vi "TrapezoidProfile_Position_Control_Example.vi"() -> ()   [LabVIEW 2019]
uses:
  <vilib>/Rock Robotics/WPI/ThirdParty/JAS_Junk/TrajLib/TrapProfile_Calculate.vi
  <vilib>/Rock Robotics/WPI/ThirdParty/JAS_Junk/TrajLib/TrapProfile_New.vi
  <vilib>/Rock Robotics/WPI/ThirdParty/JAS_Junk/TrajLib/TrapProfile_TotalTime.vi
  <vilib>/Rock Robotics/WPI/ThirdParty/JAS_Junk/TrajLib/TrapProfConstraint_New.vi
  <vilib>/Rock Robotics/WPI/ThirdParty/JAS_Junk/TrajLib/TrapProfState_New.vi
  <vilib>/Rock Robotics/WPI/ThirdParty/JAS_Junk/TrajLib/TrapProfile_IsFinished.vi
  <vilib>/Rock Robotics/WPI/ThirdParty/JAS_Junk/TrajLib/SimpleMotorFF_Calculate.vi
  <vilib>/Rock Robotics/WPI/ThirdParty/JAS_Junk/TrajLib/TrapProfile_Direct.vi
  <vilib>/Rock Robotics/WPI/ThirdParty/JAS_Junk/TrajLib/TrapProfile_ShouldFlipAcceleration.vi
  <vilib>/Rock Robotics/SystemInterfaces/NetworkCommunication/NetComm_UsageReport_report.vi
  <vilib>/Rock Robotics/WPI/ThirdParty/JAS_Junk/TrajLib/Util_LibraryGlobals.vi
  <vilib>/Rock Robotics/WPI/ThirdParty/JAS_Junk/TrajLib/Trajectory_Library.lvlib
panel:
  in  "Tab Control":T1(tab)
  out "Speed Chart":T2(graph)
  in  "Desired Position\nFt":dbl(slide) min=0.0 max=90.0 scale=-50.0..50.0
  in  "Set Desired \nPosition to \n0 Ft":bool
  in  "Set Desired \nPosition to\n15 ft":bool
  in  "Turn on to\nuse slider\nas setpoint":bool
  out "Position Error":dbl format="%14.2f"
  out "SP, PV, CO Chart":T3(graph)
  out "In Position":bool
  out "Motor-Demand":dbl format="%14.3f"
  out "Position\nFt":dbl format="%14.2f"
  out "Setpoint\nFt":dbl format="%14.2f"
  out "Velocity Ft/Sec":dbl format="%16.1f"
  out "Velocity SP Ft/Sec":dbl format="%16.1f"
  in  "Max Accel":dbl=7.0 format="%#_13g"
  # "Example of Using Trapezoid Profile for Position Control"
  # "Simulate a robot driving forward to a particular position.  A function generator is used to calculate the desired\nmotor output based on the position error.  The maximum robot speed is 8 ft/sec."
  # "Press one of the buttons \nto set the desired position.  \nThis \"target\" value is \ncalledthe \"Set Point\"."
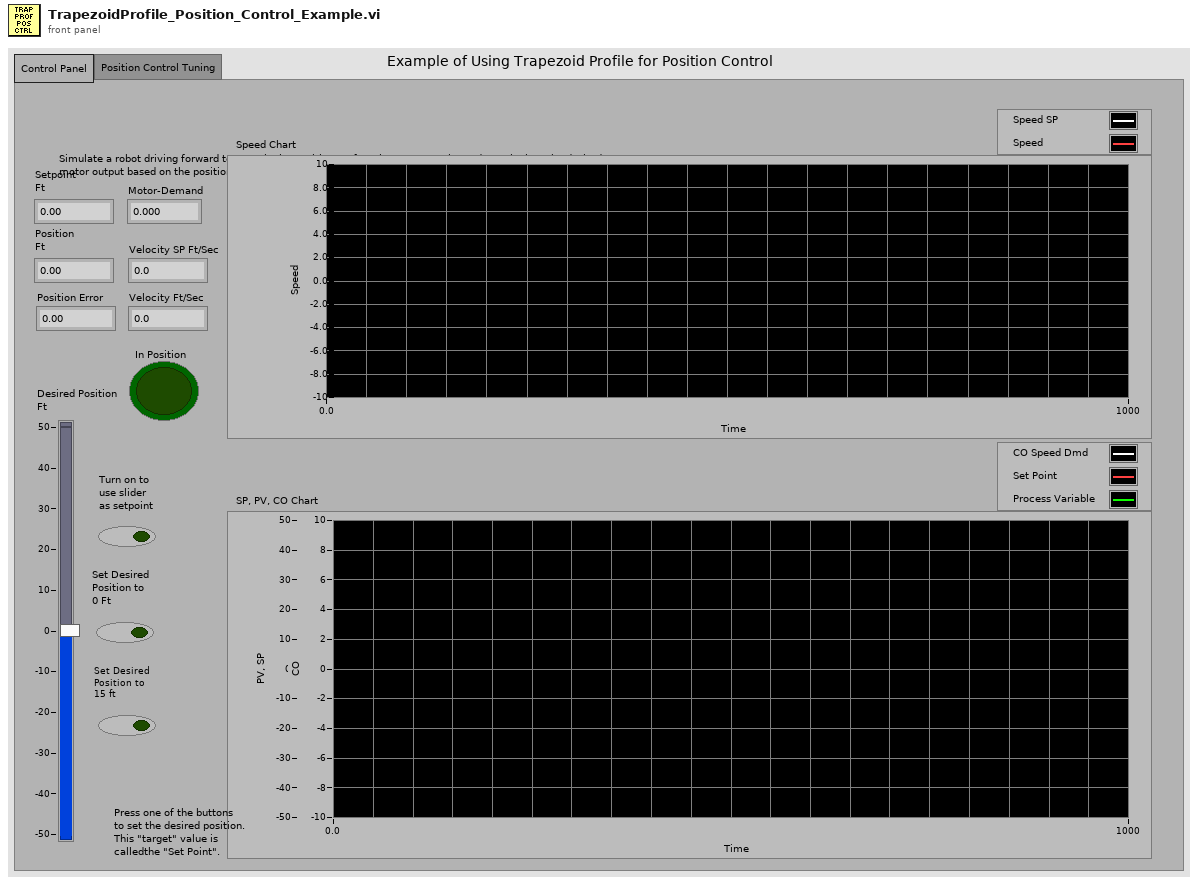
[diagram p1: front panel]
types:
  T1 = enum32{"Control Panel", "Position Control Tuning"}
  T2 = cluster{"Velocity SP Ft/Sec":dbl, "Velocity Ft/Sec":dbl}
  T3 = cluster{"MotorDemand":dbl, "CurrentSetpoint":dbl, "CurrentPosition":dbl}
  T4 = cluster{"Velocity SP Ft/Sec":dbl, "Setpoint\nFt":dbl, "Position\nFt":dbl}
  T5 = typedef "Trajectory_Library.lvlib/SIMPLE_MOTOR_FF.ctl" = cluster{"Ks":dbl, "Kv":dbl, "Ka":dbl, "KnInv":dbl}
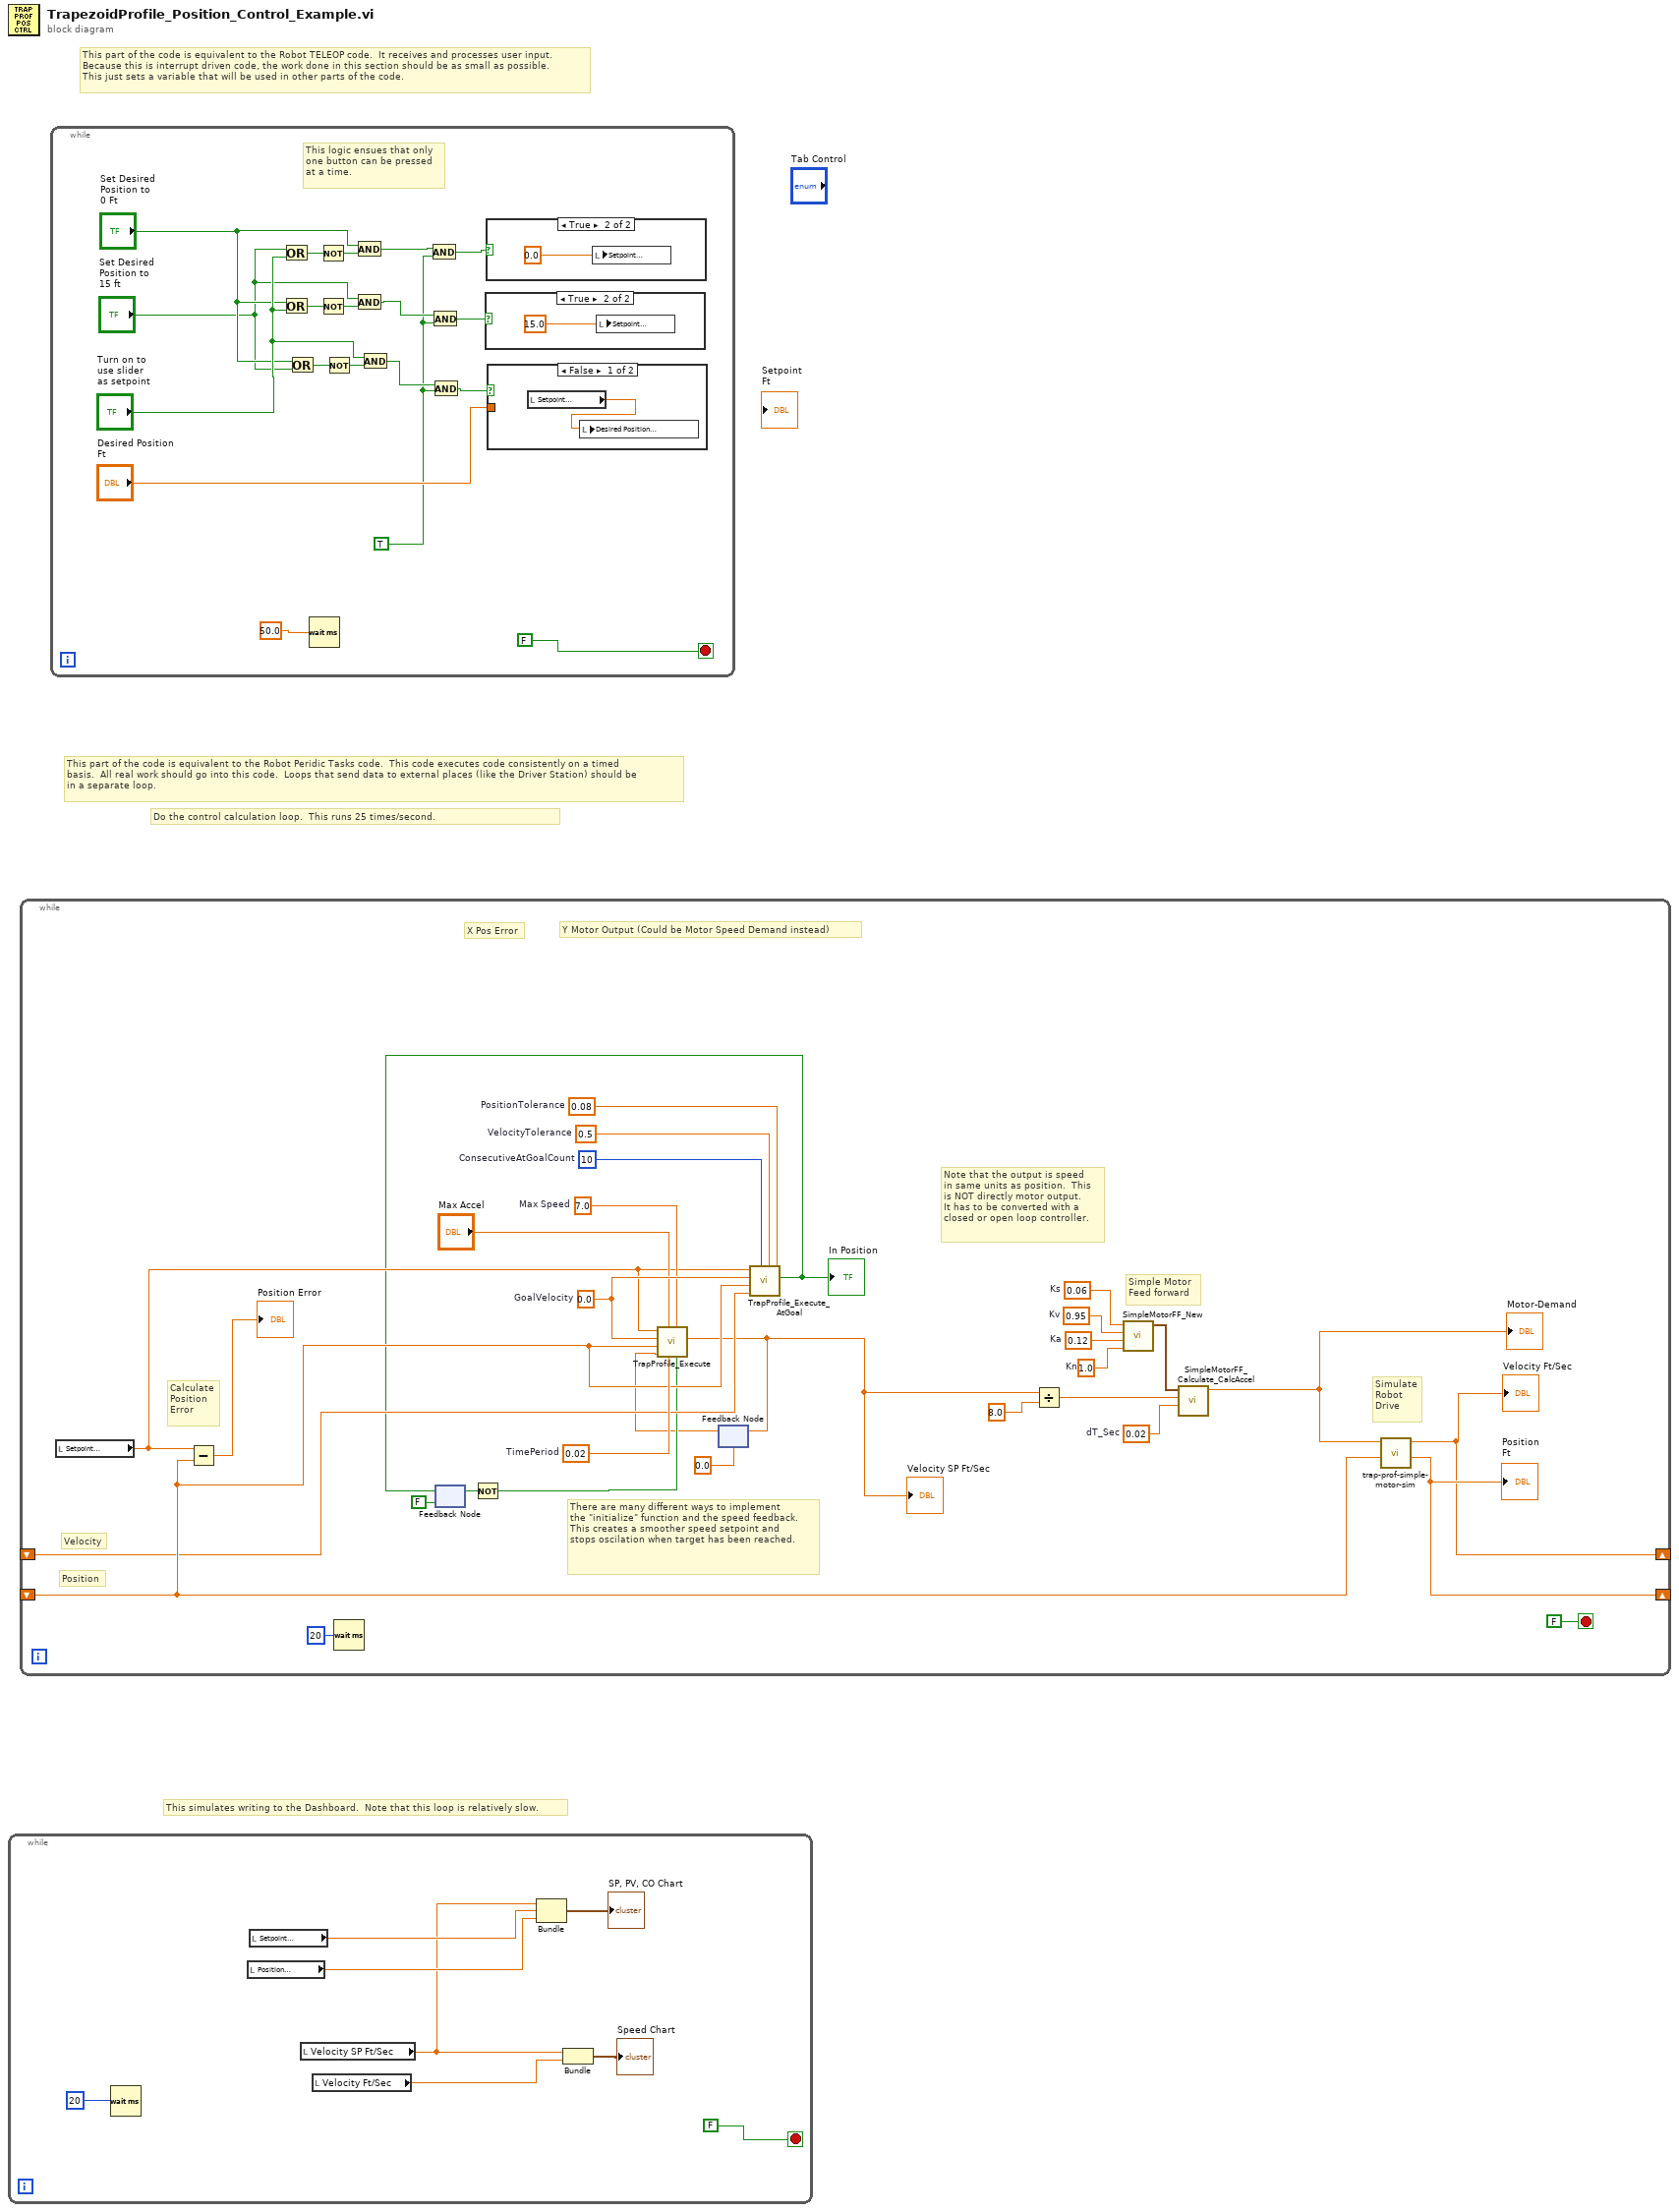
[diagram p0: block diagram]
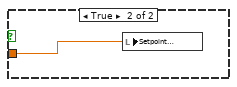
[diagram p2: hidden frame]
diagram:
  # "This simulates writing to the Dashboard.  Note that this loop is relatively slow."
  # "Do the control calculation loop.  This runs 25 times/second."
  # "This part of the code is equivalent to the Robot Peridic Tasks code.  This code executes code consistently on a timed\nbasis.  All real work should go into this code.  Loops that send data to external places (like the Driver Station) should be \nin a separate loop."
  # "This part of the code is equivalent to the Robot TELEOP code.  It receives and processes user input.\nBecause this is interrupt driven code, the work done in this section should be as small as possible.\nThis just sets a variable that will be used in other parts of the code."
  n1 = while {
    stop <- FALSE stop-if-true
    n2 = Wait (ms)(milliseconds to wait=u32 20) -> ()  [unwired: 1 out]
    n3 = local read "Position\nFt"() -> (w4:dbl)
    n4 = local read "Setpoint\nFt"() -> (w6:dbl)
    n5 = local read "Velocity SP Ft/Sec"() -> (w1:dbl)
    n6 = local read "Velocity Ft/Sec"() -> (w3:dbl)
    n7 = Bundle("Velocity SP Ft/Sec"=w1, "Setpoint\nFt"=w6, "Position\nFt"=w4) -> (→"SP, PV, CO Chart":T4)  [unwired: 1 in]
    n8 = Bundle("Velocity SP Ft/Sec"=w1, "Velocity Ft/Sec"=w3) -> (→"Speed Chart":T2)  [unwired: 1 in]
  }
  n9 = while {
    shift-right: [w37] -> _
    shift-left: _ -> [w28]
    shift-right: [w29] -> _
    shift-left: _ -> [w27]
    stop <- FALSE stop-if-true
    w24 = 1.0  # Kn
    w23 = 0.02  # dT_Sec
    w21 = 0.06  # Ks
    w20 = 0.95  # Kv
    w19 = 0.12  # Ka
    w34 = 10  # ConsecutiveAtGoalCount
    w35 = 0.5  # VelocityTolerance
    w36 = 0.08  # PositionTolerance
    w33 = 0.0  # GoalVelocity
    w31 = 0.02  # TimePeriod
    w32 = 7.0  # Max Speed
    # "Velocity"
    # "Position"
    # "Simple Motor\nFeed forward"
    # "Note that the output is speed\nin same units as position.  This\nis NOT directly motor output.\nIt has to be converted with a \nclosed or open loop controller."
    # "There are many different ways to implement\nthe \"initialize\" function and the speed feedback.\nThis creates a smoother speed setpoint and\nstops oscilation when target has been reached."
    # "Y Motor Output (Could be Motor Speed Demand instead)"
    # "X Pos Error"
    # "Calculate\nPosition\nError"
    # "Simulate\nRobot\nDrive"
    n10 = local read "Setpoint\nFt"() -> (w25:dbl)
    n11 = Subtract(x=w25, y=w28) -> (x-y=→"Position Error":dbl)
    n12 = Wait (ms)(milliseconds to wait=u32 20) -> ()  [unwired: 1 out]
    n13 = feedback #1(FALSE ("AtGoal")) -> (w14:bool)
    n14 = Not(x=w14) -> (.not. x?=w13:bool)
    n15 = feedback #2(0.0 ("VelocityDmd")) -> (w11:dbl)
    n16 = call <vilib>:"TrapProfile_Execute.vi"("Initialize"=w13, "Max Speed"=w32, "TimePeriod"=w31, "Max Accel"="Max Accel", "CurrentVelocity"=w11, "CurrentPosition"=w28, "GoalVelocity"=w33, "GoalPosition"=w25) -> ("VelocityDmd"=w12:dbl)  [unwired: 3 out]
    "Velocity SP Ft/Sec" <- w12
    n17 = feedback-in #2(w12) -> ()
    n18 = call <vilib>:"TrapProfile_Execute_AtGoal.vi"("PositionTolerance"=w36, "VelocityTolerance"=w35, "ConsecutiveAtGoalCount"=w34, "CurrentVelocity"=w27, "CurrentPosition"=w28, "GoalVelocity"=w33, "GoalPosition"=w25) -> ("AtGoal"=w16:bool)  [unwired: 4 in]
    "In Position" <- w16
    n19 = feedback-in #1(w16) -> ()
    n20 = Divide(x=w12, y=8.0) -> (x/y=w18:dbl)
    n21 = call <vilib>:"SimpleMotorFF_New.vi"("Kn"=w24, "Ka"=w19, "Kv"=w20, "Ks"=w21) -> ("SIMPLE_MOTOR_FF"=w22:T5)  [unwired: 7 in]
    n22 = call <vilib>:"SimpleMotorFF_Calculate_CalcAccel.vi"("dT_Sec"=w23, "VelSp"=w18, "SIMPLE_MOTOR_FF"=w22) -> ("FeedForward"=w17:dbl)  [unwired: 8 in]
    "Motor-Demand" <- w17
    n23 = call "trap-prof-simple-motor-sim.vi"("Current Position Ft"=w28, "Motor-Demand"=w17) -> ("Updated Position Ft"=w37:dbl, "Velocity Ft/Sec"=w29:dbl)  [unwired: 8 in]
    "Position\nFt" <- w37
    "Velocity Ft/Sec" <- w29
  }
  n24 = while {
    stop <- FALSE stop-if-true
    w40 = TRUE
    # "This logic ensues that only\none button can be pressed\nat a time."
    n25 = Or(x="Set Desired \nPosition to\n15 ft", y="Turn on to\nuse slider\nas setpoint") -> (x .or. y?=w58:bool)
    n26 = Or(x="Set Desired \nPosition to \n0 Ft", y="Turn on to\nuse slider\nas setpoint") -> (x .or. y?=w56:bool)
    n27 = Or(x="Set Desired \nPosition to \n0 Ft", y="Set Desired \nPosition to\n15 ft") -> (x .or. y?=w54:bool)
    n28 = Wait (ms)(milliseconds to wait=50.0) -> ()  [unwired: 1 out]
    n29 = Not(x=w58) -> (.not. x?=w57:bool)
    n30 = Not(x=w56) -> (.not. x?=w55:bool)
    n31 = Not(x=w54) -> (.not. x?=w53:bool)
    n32 = And(x="Set Desired \nPosition to \n0 Ft", y=w57) -> (x .and. y?=w49:bool)
    n33 = And(x="Set Desired \nPosition to\n15 ft", y=w55) -> (x .and. y?=w45:bool)
    n34 = And(x="Turn on to\nuse slider\nas setpoint", y=w53) -> (x .and. y?=w44:bool)
    n35 = And(x=w49, y=w40) -> (x .and. y?=w48:bool)
    n36 = And(x=w45, y=w40) -> (x .and. y?=w47:bool)
    n37 = And(x=w44, y=w40) -> (x .and. y?=w46:bool)
    n38 = case shown="True" w47 {
      frame False {
      }
      frame True {
        n39 = local write "Setpoint\nFt"(15.0) -> ()
      }
    }
    n40 = case shown="True" w48 {
      frame False {
      }
      frame True {
        n41 = local write "Setpoint\nFt"(0.0) -> ()
      }
    }
    n42 = case shown="False" w46 {
      tunnel: "Desired Position\nFt" -> [_ w60]
      frame False {
        n43 = local read "Setpoint\nFt"() -> (w59:dbl)
        n44 = local write "Desired Position\nFt"(w59) -> ()
      }
      frame True {
        n45 = local write "Setpoint\nFt"(w60) -> ()
      }
    }
  }
